vi "Check Rate.vi"(1 "Rate":dbl format="%.2f", 2 "Field":dbl format="%.2f", 3 "input cluster":T1 {"MaxLambdaCurrent [A]" format="%.2f"; "LambdaRates [A/min]" format="%.2f"; "MaxNormalCurrent [A]" format="%.2f"; "StabilitySetting [%]" format="%.2f"; "FieldCurrentRatio [T/A]" format="%.2f"; "SwitchWaitTime [s]" format="%.2f"; "SwitchHtrCurrent [mA]" format="%.2f"; "TrainRates [A/min]" format="%.2f"; "NormalRates [A/min]" format="%.2f"; "Breakpts [A]" format="%.2f"}) -> (0 "Checked Rate":dbl format="%.6f")   [LabVIEW 2019]
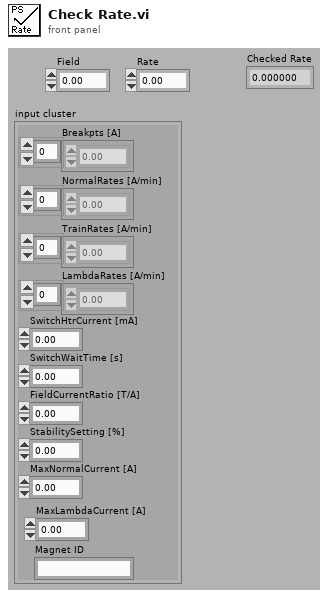
[diagram p1: front panel]
types:
  T1 = cluster{"Breakpts [A]":dbl[], "NormalRates [A/min]":dbl[], "TrainRates [A/min]":dbl[], "SwitchHtrCurrent [mA]":dbl, "SwitchWaitTime [s]":dbl, "FieldCurrentRatio [T/A]":dbl, "StabilitySetting [%]":dbl, "MaxNormalCurrent [A]":dbl, "Magnet ID":string, "LambdaRates [A/min]":dbl[], "MaxLambdaCurrent [A]":dbl}
  T2 = enum16{"Normal", "Train", "Lambda", "Train & Lambda"}
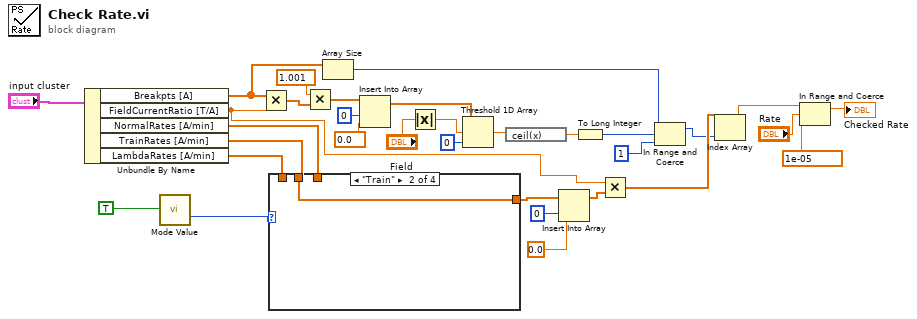
[diagram p0: block diagram]
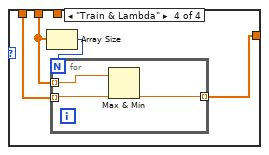
[diagram p4: hidden frame]
diagram:
  n1 = Unbundle By Name("input cluster") -> ("Breakpts [A]"=w25:dbl[], "FieldCurrentRatio [T/A]"=w23:dbl, "NormalRates [A/min]"=w20:dbl[], "TrainRates [A/min]"=w21:dbl[], "LambdaRates [A/min]"=w16:dbl[])
  n2 = call "Mode Value.vi"("Read/Write this vi"=TRUE) -> ("Mode Out"=w18:T2)  [unwired: 1 in]
  n3 = Multiply(x=w25, y=w23) -> (x*y=w31:dbl[])
  n4 = case shown="\"Train\"" w18 {
    tunnel: w21 -> [_ w34 _ w38]
    tunnel: w20 -> [w33 _ _ _]
    tunnel: [w33 w34 w35 w36] -> w19
    tunnel: w16 -> [_ _ w35 w37]
    frame "Normal", Default {
    }
    frame "Train" {
    }
    frame "Lambda" {
    }
    frame "Train & Lambda" {
      n5 = Array Size(array=w38) -> (size(s)=w39:i32)
      n6 = for {
        N: w39 -> [_]
        tunnel: w38 -> [w42] mode=indexing
        tunnel: w37 -> [w41] mode=indexing
        tunnel: [w40] -> w36 mode=indexing
        n7 = Max & Min(x=w42, y=w41) -> (min(x,y)=w40:dbl)  [unwired: 1 out]
      }
    }
  }
  n8 = Multiply(x=1.001, y=w31) -> (x*y=w2:dbl[])
  n9 = Array Size(array=w25) -> (size(s)=w7:i32)
  n10 = Insert Into Array(array=w2, index=0, new element=0.0 ("new element/subarray")) -> (w28:dbl[])
  n11 = Absolute Value(x="Field") -> (abs(x)=w13:dbl)
  n12 = Threshold 1D Array(1:0 ("start index (0)"), 2:w13, 3:w28) -> (0:w27:dbl)
  n13 = expression code="ceil(x)"(w27) -> (w6:dbl)
  n14 = Insert Into Array(array=w19, index=0, new element=0.0 ("new element/subarray")) -> (w10:dbl[])
  n15 = To Long Integer(number=w6) -> (32bit integer=w5:i32)
  n16 = Multiply(x=w23, y=w10) -> (x*y=w24:dbl[])
  n17 = In Range and Coerce(upper limit=w7, x=w5, lower limit=1) -> (coerced(x)=w3:i32)  [unwired: 1 out]
  n18 = Index Array(array=w24, index=w3) -> (element=w9:dbl)
  n19 = In Range and Coerce(upper limit=w9, x="Rate", lower limit=1e-05) -> (coerced(x)=→"Checked Rate":dbl)  [unwired: 1 out]
